vi "rqcBob KeyNET Read Data.vi"(8 "error in":errorcluster, 11 "rqcBob KeyNET in":T1) -> (0 "error out":errorcluster, 1 "data valid":bool, 2 "Data":u32[](array[numeric]), 3 "rqcBob KeyNET out":T1)   [LabVIEW 2016]
uses:
  Custom Controls/rqcBob KeyNET control.ctl
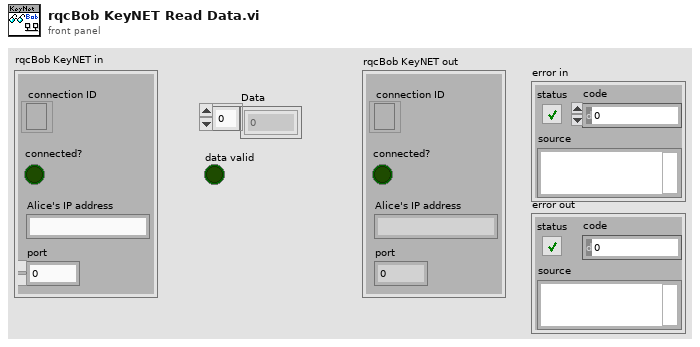
[diagram p1: front panel]
types:
  T1 = typedef "rqcBob KeyNET control.ctl" = cluster{"connection ID":refnum<k5>, "connected?":bool, "Alice's IP address":string, "port":u16}
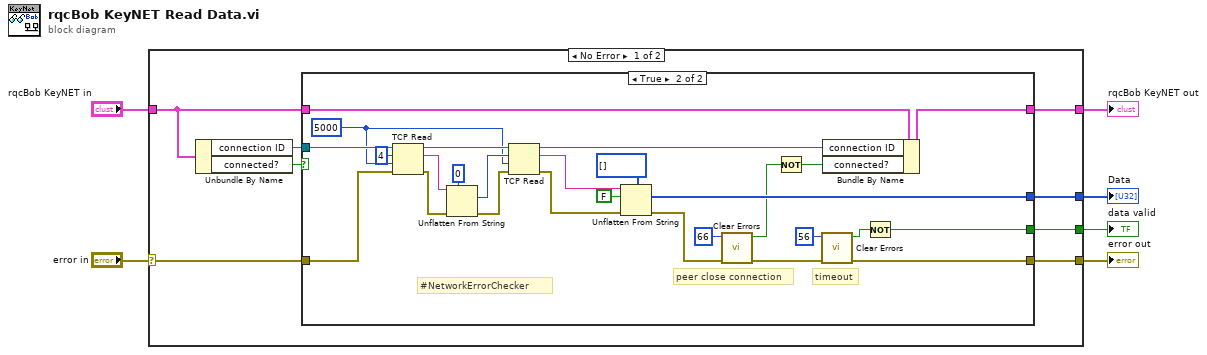
[diagram p0: block diagram]
diagram:
  n1 = case shown="No Error" "error in" {
    selector: "error in" -> [w12 w45]
    tunnel: "rqcBob KeyNET in" -> [w10 w44]
    tunnel: [w11 w45] -> w4
    tunnel: [w9 w44] -> w3
    tunnel: [w8 _] -> w2
    tunnel: [w7 _] -> w1
    frame No Error {
      n2 = Unbundle By Name(w10) -> ("connection ID"=w13:refnum<k5>, "connected?"=w14:bool)
      n3 = case shown="True" w14 {
        tunnel: w13 -> [_ w41]
        tunnel: w12 -> [w16 w40]
        tunnel: [w16 w17] -> w11
        tunnel: [w15 w42] -> w9
        tunnel: w10 -> [w15 w43]
        tunnel: [_ w27] -> w8
        tunnel: [_ w18] -> w7
        frame False {
        }
        frame True {
          w24 = 5000 ("timeout ms (25000)")
          # "peer close connection"
          # "timeout"
          # "#NetworkErrorChecker"
          n4 = TCP Read(connection ID=w41, bytes to read=4, error in (no error)=w40, 9:w24) -> (connection ID out=w35:refnum<k5>, data out=w38:string, error out=w36:errorcluster)  [unwired: 1 in]
          n5 = Unflatten From String(type=0, binary string=w38, error in (no error)=w36) -> (value=w32:i32, error out=w33:errorcluster)  [unwired: 2 in, 1 out]
          n6 = TCP Read(connection ID=w35, bytes to read=w32, error in (no error)=w33, 9:w24) -> (connection ID out=w34:refnum<k5>, data out=w30:string, error out=w31:errorcluster)  [unwired: 1 in]
          n7 = Unflatten From String(type=u32[] [], binary string=w30, data includes array or string size? (T)=FALSE, error in (no error)=w31) -> (value=w27:u32[], error out=w21:errorcluster)  [unwired: 1 in, 1 out]
          n8 = call <vilib>:"Clear Errors.vi"("error in (no error)"=w21, "specific error code to clear (0: all)"=66) -> ("error out"=w20:errorcluster, "specific error cleared?"=w23:bool)  [unwired: 4 in]
          n9 = Not(x=w23) -> (.not. x?=w22:bool)
          n10 = call <vilib>:"Clear Errors.vi"("error in (no error)"=w20, "specific error code to clear (0: all)"=56) -> ("error out"=w17:errorcluster, "specific error cleared?"=w19:bool)  [unwired: 4 in]
          n11 = Bundle By Name(cluster=w43, "connection ID"=w34, "connected?"=w22) -> (w42:T1)
          n12 = Not(x=w19) -> (.not. x?=w18:bool)
        }
      }
    }
    frame Error {
    }
  }
  "error out" <- w4
  "rqcBob KeyNET out" <- w3
  "Data" <- w2
  "data valid" <- w1
